vi "First step heating with process.vi"(0 "Arduino Resource In":T1={"VISA resource"="", "Board Type"=enum."Uno", "Connection Type"=enum."USB / Serial", "Bytes Per Packet (15)"=15}, 11 "Error In":errorcluster, 12 "shift left":i32, 13 "Запуск процесса":bool) -> (4 "Arduino Resource Out":T1={"VISA resource"="", "Board Type"=enum."Uno", "Connection Type"=enum."USB / Serial", "Bytes Per Packet (15)"=15}, 14 "Shift right":i32, 15 "Error Out":errorcluster)   [LabVIEW 2016]
uses:
  <vilib>/LabVIEW Interface for Arduino/Type Defs/Arduino Resource.ctl
  <vilib>/LabVIEW Interface for Arduino/Type Defs/Board Type.ctl
  <vilib>/LabVIEW Interface for Arduino/LabVIEW Interface for Arduino.lvlib
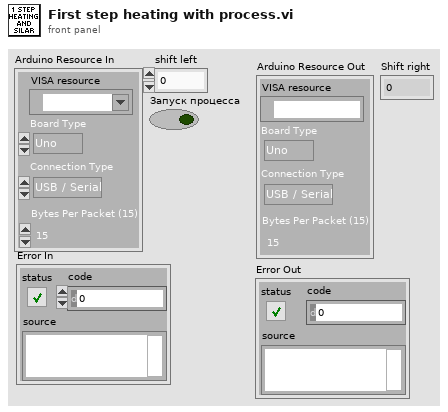
[diagram p1: front panel]
types:
  T1 = typedef "LabVIEW Interface for Arduino.lvlib/Arduino Resource.ctl" = cluster{"VISA resource":refnum<visa-resource-name>, "Board Type":T2, "Connection Type":enum8{"USB / Serial"}, "Bytes Per Packet (15)":u8}
  T2 = typedef "LabVIEW Interface for Arduino.lvlib/Board Type.ctl" = enum16{"Uno", "Dimuelanove w/Atmega 328", "Mega 2560"}
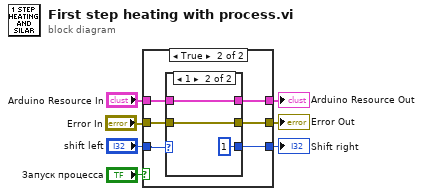
[diagram p0: block diagram]
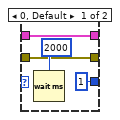
[diagram p3: hidden frame]
diagram:
  n1 = case shown="True" "Запуск процесса" {
    tunnel: "Error In" -> [w9 w16]
    tunnel: [w9 w15] -> w1
    tunnel: "Arduino Resource In" -> [w10 w13]
    tunnel: [w10 w14] -> w2
    tunnel: [w8 w12] -> w3
    tunnel: "shift left" -> [w8 w11]
    frame False {
    }
    frame True {
      n2 = case shown="1" w11 {
        tunnel: w16 -> [w19 w22]
        tunnel: [w19 w22] -> w15
        tunnel: [w18 w23] -> w14
        tunnel: w13 -> [w18 w23]
        tunnel: [1 1] -> w12
        frame 0, Default {
          n3 = Wait (ms)(milliseconds to wait=u32 2000) -> ()  [unwired: 1 out]
        }
        frame 1 {
        }
      }
    }
  }
  "Shift right" <- w3
  "Arduino Resource Out" <- w2
  "Error Out" <- w1
